vi "KE_scan_Init.vi"(4 "error in (no error)":errorcluster, 6 "GPIB (t) / RS-232 (f)":bool, 8 "Current Range Ch 2":T1 items=["Autorange", "+/- 20 mikroA", "+/- 2 mikroA", "+/- 200 nA", "+/- 20 nA", "+/- 2 nA"], 9 "Current Range Ch 1":T1 items=["Autorange", "+/- 20 mikroA", "+/- 2 mikroA", "+/- 200 nA", "+/- 20 nA", "+/- 2 nA"], 10 "Cluster":T2={"Baudrate (9600)"=57600, "Data Bits (8)"=8, "Parity (None)"=0, "Stop Bits (1)"=10, "Flow Control (None)"=0, "End Mode for Reads (TermChar)"=2} {"End Mode for Reads (TermChar)" items=["None", "Last Bit", "TermChar"]; "Flow Control (None)" items=["None", "XON/XOFF", "RTS/CTS", "XON/XOFF & RTS/CTS", "DTR/DSR", "XON/XOFF & DTR/DSR"]; "Stop Bits (1)" items=["1.0"=10, "1.5"=15, "2.0"=20]; "Parity (None)" items=["None", "Odd", "Even", "Mark", "Space"]; "Baudrate (9600)" items=["9600"=9600, "19200"=19200, "38400"=38400, "57600"=57600, "115200"=115200]}, 11 "Address in":refnum<visa-resource-name>="GPIB0::25::INSTR") -> (0 "error out":errorcluster, 3 "VISA resource name out":refnum<visa-resource-name>)   [LabVIEW 2018]
uses:
  Keithley Picoammeter/subVIs/Current_Range_Control.ctl
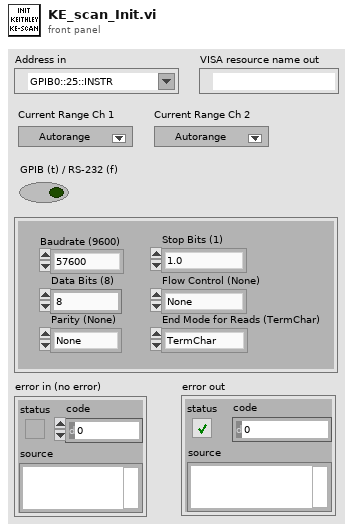
[diagram p1: front panel]
types:
  T1 = typedef "Current_Range_Control.ctl" = u16
  T2 = cluster{"Baudrate (9600)":u32, "Data Bits (8)":u16, "Parity (None)":u16, "Stop Bits (1)":u16, "Flow Control (None)":u16, "End Mode for Reads (TermChar)":u16}
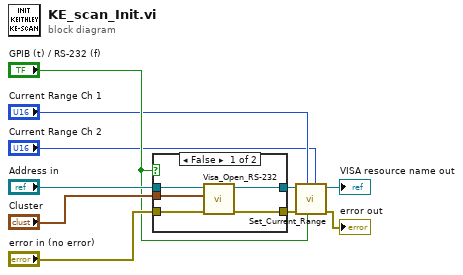
[diagram p0: block diagram]
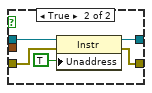
[diagram p2: hidden frame]
diagram:
  n1 = case shown="False" "GPIB (t) / RS-232 (f)" {
    tunnel: "Address in" -> [w15 w19]
    tunnel: "error in (no error)" -> [w12 w18]
    tunnel: [w14 w17] -> w7
    tunnel: [w13 w16] -> w6
    tunnel: "Cluster" -> [w11 _]
    frame False {
      n2 = call "Visa_Open_RS-232.vi"("error in (no error)"=w12, "Cluster"=w11, "ComPort"=w15) -> ("error out"=w13:errorcluster, "VISA resource name out"=w14:refnum<visa-resource-name>)  [unwired: 7 in]
    }
    frame True {
      n3 = property class="Instr"(reference=w19, error in=w18, "Unaddress"=TRUE ("GPIB Settings:Unaddressing")) -> (reference out=w17:refnum<visa-resource-name>, error out=w16:errorcluster)
    }
  }
  n4 = call "Set_Current_Range.vi"("Current Range Ch 2"="Current Range Ch 2", "GPIB (t) / RS-232 (f)"="GPIB (t) / RS-232 (f)", "Current Range Ch 1"="Current Range Ch 1", "error in (no error)"=w6, "VISA resource name"=w7) -> ("error out"=→"error out":errorcluster, "VISA resource name out"=→"VISA resource name out":refnum<visa-resource-name>)  [unwired: 5 in]
